vi "PZT init.vi"(2 "error in (no error)":errorcluster caption="错误输入（无错误）", 3 "Ch":enum16{"CH1", "CH2", "CH3"}(ring), 4 "Communication":enum16{"USB", "LAN"}(ring), 5 "VISA resource name":refnum<visa-resource-name> caption="VISA资源名称") -> (0 "错误输出":errorcluster, 1 "VISA资源名称输出":refnum<visa-resource-name>)   [LabVIEW 2019]
uses:
  <vilib>/Instr/_visa.llb/VISA Configure Serial Port (Instr).vi
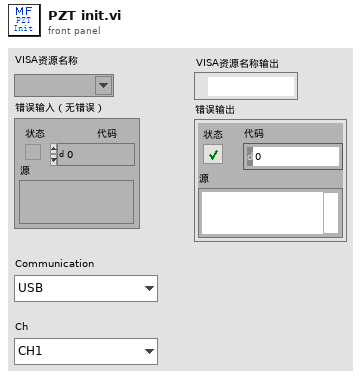
[diagram p1: front panel]
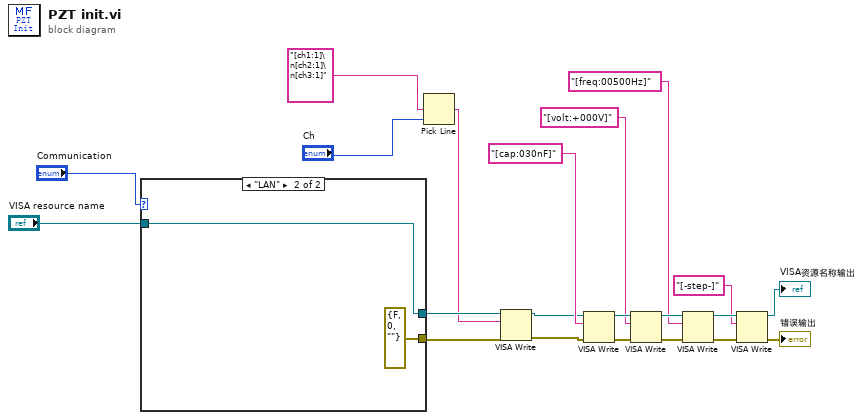
[diagram p0: block diagram]
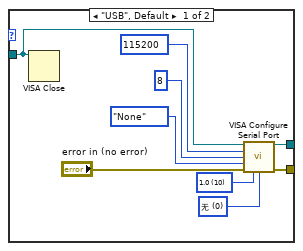
[diagram p2: hidden frame]
diagram:
  n1 = case shown="\"LAN\"" "Communication" {
    tunnel: [w26 w32] -> w7
    tunnel: [w23 errorcluster {"status"=FALSE, "code"=0, "source"=""} ("error out")] -> w6
    tunnel: "VISA resource name" -> [w22 w32]
    frame "USB", Default {
      w24 = u16 0 items=["无", "XON/XOFF", "RTS/CTS", "XON/XOFF & RTS/CTS", "DTR/DSR", "XON/XOFF & DTR/DSR"] ("flow control (0:none)")
      w27 = u16 10 items=["1.0"=10, "1.5"=15, "2.0"=20] ("stop bits (10: 1 bit)")
      n2 = VISA Close(VISA resource name=w22) -> ()  [unwired: 1 in, 1 out]
      n3 = call-poly "VISA Configure Serial Port"("VISA resource name"=w22, "baud rate (9600)"=u32 115200, "data bits (8)"=u16 8, "parity (0:none)"=enum16{"None", "Odd", "Even", "Mark", "Space"}."None", "error in (no error)"="error in (no error)", "stop bits (10: 1 bit)"=w27, "flow control (0:none)"=w24) -> ("VISA resource name out"=w26:refnum<visa-resource-name>, "error out"=w23:errorcluster)  [unwired: 7 in]
    }
    frame "LAN" {
    }
  }
  n4 = Pick Line(multi-line string="[ch1:1]\n[ch2:1]\n[ch3:1]" ("写入缓冲区"), line index="Ch") -> (output string=w2:string)  [unwired: 1 in]
  n5 = VISA Write(VISA resource name=w7, write buffer=w2, error in (no error)=w6) -> (VISA resource name out=w5:refnum<visa-resource-name>, error out=w4:errorcluster)  [unwired: 1 out]
  n6 = VISA Write(VISA resource name=w5, write buffer="[cap:030nF]" ("写入缓冲区"), error in (no error)=w4) -> (VISA resource name out=w20:refnum<visa-resource-name>, error out=w13:errorcluster)  [unwired: 1 out]
  n7 = VISA Write(VISA resource name=w20, write buffer="[volt:+000V]" ("写入缓冲区"), error in (no error)=w13) -> (VISA resource name out=w19:refnum<visa-resource-name>, error out=w12:errorcluster)  [unwired: 1 out]
  n8 = VISA Write(VISA resource name=w19, write buffer="[freq:00500Hz]" ("写入缓冲区"), error in (no error)=w12) -> (VISA resource name out=w16:refnum<visa-resource-name>, error out=w11:errorcluster)  [unwired: 1 out]
  n9 = VISA Write(VISA resource name=w16, write buffer="[-step-]" ("写入缓冲区"), error in (no error)=w11) -> (VISA resource name out=→"VISA资源名称输出":refnum<visa-resource-name>, error out=→"错误输出":errorcluster)  [unwired: 1 out]
